vi "pump rpm cluster.vi"() -> (2 "pump speed":dbl[unit] format="%.2f", 3 "pump speed (rpm)":dbl format="%.2f", 4 "tube diameter":dbl[unit] format="%.2f", 5 "in range":bool)   [LabVIEW 2010]
uses:
  Stamp/calibration commands.ctl
panel:
  in  "Pump":T1 {"flow rate" format="%.2f"}
  in  "diameter":dbl[unit][](array[numeric])=[0.00079375, 0.0015875, 0.003175, 0.004762499999999999, 0.00635, 0.0079375] format="%.5f"
  in  "pumpflow":dbl[unit][](array[numeric])=[9.549296547316535e-09, 3.342253804929783e-08, 1.2732395447351617e-07, 2.705634032562094e-07, 4.4563384065730255e-07, 6.04788783748884e-07] format="%.3f"
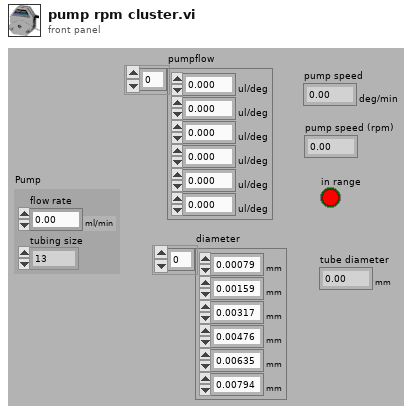
[diagram p1: front panel]
types:
  T1 = cluster{"tubing size":enum16{"13", "14", "16", "25", "17", "18"}, "flow rate":dbl[unit]}
  T2 = typedef "calibration commands.ctl" = enum16{"Get ini Path", "Save default values", "Save new calibration", "Read calibration", "Apply calibration", "Read STAMP mb", "Write STAMP mb"}
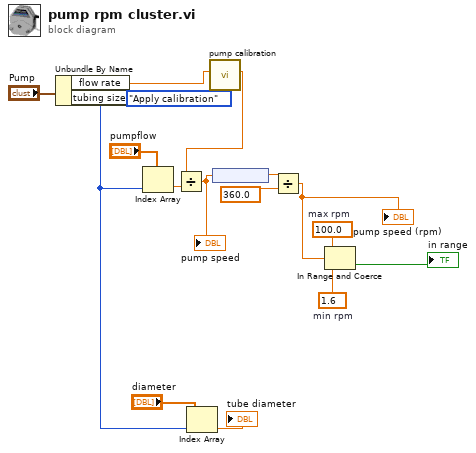
[diagram p0: block diagram]
diagram:
  w8 = 1.6  # min rpm
  w9 = 100.0  # max rpm
  n1 = Unbundle By Name("Pump") -> ("flow rate"=w2:dbl[unit], "tubing size"=w4:enum16{"13", "14", "16", "25", "17", "18"})
  n2 = Index Array(array="pumpflow", index=w4) -> (element=w15:dbl[unit])
  n3 = Index Array(array="diameter", index=w4) -> (element=→"tube diameter":dbl[unit])
  n4 = call "pump calibration.vi"("pump cal command"=calibration_commands."Apply calibration", "flow rate"=w2) -> ("modified flow rate"=w1:dbl[unit])  [unwired: 3 in, 3 out]
  n5 = Divide(x=w1, y=w15) -> (x/y=w14:dbl[unit])
  "pump speed" <- w14
  n6 = node(w14) -> (w13:dbl)
  n7 = Divide(x=w13, y=360.0) -> (x/y=w6:dbl)
  "pump speed (rpm)" <- w6
  n8 = In Range and Coerce(upper limit=w9, x=w6, lower limit=w8) -> (In Range?=→"in range":bool)  [unwired: 1 out]
